vi "AlliGator Compute Pixel Phasor Array v3.vi"(6 "e^j w t_i Vector":csg[](array[numeric]), 7 "Time-Gated Reference Decay":cluster{"t Array":dbl[], "I Array":dbl[]}, 8 "Error In":errorcluster, 9 "t Array":sgl[](array[numeric]), 10 "Gate Images Stack (NxVxH)":sgl[][][](array[numeric]), 11 "Sum Image (V x H)":sgl[][](array[numeric])) -> (0 "Error Out":errorcluster, 1 "# Invalid Phasors":i32, 3 "Pixel Phasors Array (V x H)":csg[][](array[numeric]) format="%_3e", 4 "CPU (s)":dbl)   [LabVIEW 2021, in "AlliGator Phasor Plot.lvlib"]
doc: "Computes the phasor of all pixels using any user-selected decay pre-processing options."
uses:
  AlliGator Phasor Plot.lvlib
  Settings/AlliGator Settings List.ctl
  Globals, Variables, Constants/AlliGator Abort.vi
  <vilib>/Utility/error.llb/Error Cluster From Error Code.vi
  <vilib>/ErrorRing/Error Ring.xnode
  Time/Time.lvlib
  Phasor/Phasor.lvlib
  Graphs/XY Graph/XY Graph Add-Ons.lvlib
  Decay Analysis/Decay Preprocessing/AlliGator Decay Preprocessing.lvlib
  Globals, Variables, Constants/AlliGator Globals, Variables & Constants.lvlib
  Settings/AlliGator Settings.lvlib
  Error/Error.lvlib
  Utilities/Utilities.lvlib
panel:
  out "Local Error":errorcluster
  # "see the AlliGator License on the block diagram (Ctrl+E or Window:Show Block Diagram)"
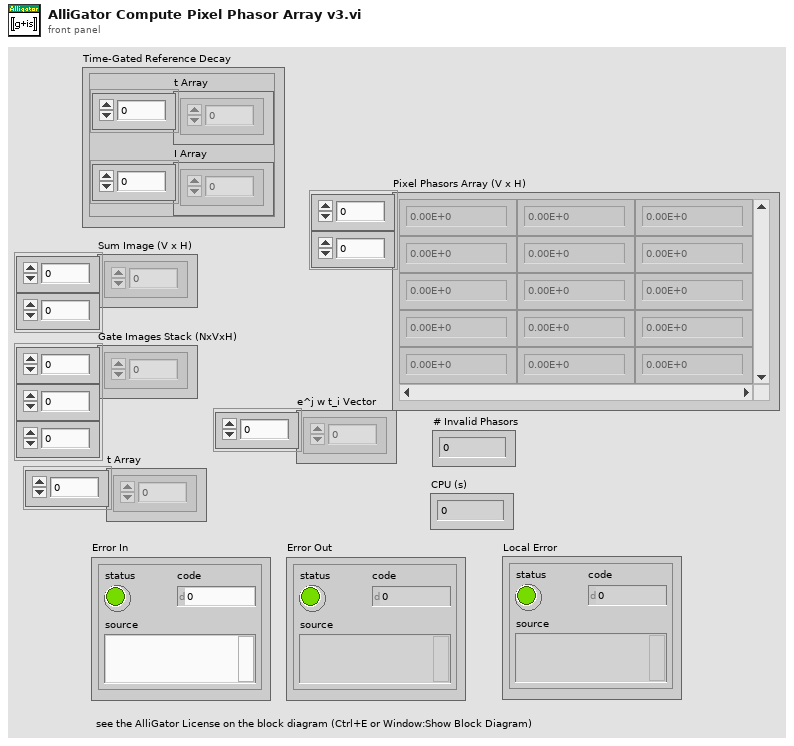
[diagram p1: front panel]
types:
  T1 = typedef "AlliGator Settings.lvlib/AlliGator Settings List.ctl" = enum16{"GUI:Visible Settings Tab", "GUI:Last Run Version", "Source Image:Use Image Histogram for Contrast", "Source Image:Low Count Pixels Rejection Options", "Source Image:High Count Pixels Rejection Options", "Source Image:Use Image Brightness", "Source Image:Blend Overlay with Image Background", "Source Image:Use Fixed ROI Diameter", "Source Image:ROI Diameter", "Source Image:ROI Center Color", "Source Image:Peak Threshold", "Source Image:Intensity Threshold", "Source Image:Image Binning Options", "Source Image:Image Smoothing Options", "Source Image:Image Histogram Active", "Source Image:Invert Binary Mask", "Source Image:Hot Pixel Removal", "Source Image:Overlay Analyzed ROI Center", "Source Image:Auto-Adjust Contrast", "Source Image:Histogram Lower Percentile", "Source Image:Histogram Upper Percentile", "Source Image:Save Source Image", "Source Image:Scale Bar Options", "Source Image:Image Resolution (Pixel Size)", "Source Image:Flatfield Correction", "Source Image:Show Dead Left Columns Correction", "Source Image:Dead Left Columns Correction", "Source Image:Image Pre-Processing Operations Order", "Source Image:Overlay ROI Median", "Source Image:Median Overlay Color", "Data Information:Gate Width", "Data Information:Nanotime Gate Separation", "Data Information:Macrotime Gate Separation", "Data Information:Gate Step", "Data Information:# Gates", "Data Information:Gate Image Exposure", "Data Information:Gate Image Integration", "Data Information:Gates to Skip", "Data Information:Gates to Keep", "Data Information:Define Gates to", "Data Information:Channel Name", "Data Information:Available Channel Names", "Data Information:Channel Arithmetic", "Data Information:Background File Subtraction", "Data Information:Background File", "Data Information:Background Scaling Factor", "Data Information:Background Pile-up Correction", "Data Information:Background Pixel Well Capacity", "Data Information:Laser Period", "Data Information:SYNC Period", "Data Information:Pile-up Correction", "Data Information:Pixel Well Capacity", "Data Information:Dataset Scaling Factor", "Fluorescence Decay_Decay Pre-Processing:Reverse Gates", "Fluorescence Decay_Decay Pre-Processing:Verbose Decay Pre-Processing", "Fluorescence Decay_Decay Pre-Processing:Use Decay Pre-Processing", "Fluorescence Decay_Decay Pre-Processing:Background Subtraction", "Fluorescence Decay_Decay Pre-Processing:Background Definition Range", "Fluorescence Decay_Decay Pre-Processing:Baseline Subtraction Method", "Fluorescence Decay_Decay Pre-Processing:Decay Pre-Processing Operations Order", "Fluorescence Decay_Decay Pre-Processing:Smoothing Parameter", "Fluorescence Decay_Decay Pre-Processing:Shift Decay", "Fluorescence Decay_Decay Pre-Processing:Decay Shift Parameters", "Fluorescence Decay_Decay Pre-Processing:Fold Decay", "Fluorescence Decay_Decay Pre-Processing:# Folds", "Fluorescence Decay_Decay Pre-Processing:1-Normalize Decay", "Fluorescence Decay_Decay Pre-Processing:[0-1]-Normalize Decay", "Fluorescence Decay_Decay Pre-Processing:Smoothen Decay", "Fluorescence Decay_Decay Pre-Processing:Extrapolate Decay", "Fluorescence Decay_Decay Pre-Processing:Use Periodicity", "Fluorescence Decay_Decay Pre-Processing:Use Cursors", "Fluorescence Decay_Decay Pre-Processing:Tail Fraction", "Fluorescence Decay_Decay Pre-Processing:Head Fraction", "Fluorescence Decay_Decay Pre-Processing:Additional Points", "Fluorescence Decay_Decay Pre-Processing:Straighten Decay", "Fluorescence Decay_Decay Pre-Processing:Constant Background", "Fluorescence Decay_Decay Pre-Processing:Pixel-Normalize Decay", "Fluorescence Decay_Advanced Analysis:Extract IRF instead of Decay", "Fluorescence Decay_Advanced Analysis:IRF Extraction Options", "Fluorescence Decay_Advanced Analysis:IRF Optimization Options", "Fluorescence Decay_Advanced Analysis:Square Pulse Options", "Fluorescence Decay_Advanced Analysis:IRF Order", "Fluorescence Decay_Advanced Analysis:IRF Time Constants", "Fluorescence Decay_Advanced Analysis:Wavelet Analysis Options", "Fluorescence Decay_Advanced Analysis:Average Lifetime Options", "Fluorescence Decay_Fit Options:Fit Options", "Fluorescence Decay_Fit Options:Use Legacy Fitting Approach", "Fluorescence Decay_Fit Options:Use Data Information Laser Period", "Fluorescence Decay_Fit Parameters:Displayed Fit Parameters", "Fluorescence Decay_Fit Parameters:Fit Parameter Constraints", "Fluorescence Decay_Fit Parameters:Export Tabulated Results", "Fluorescence Decay_Fit Parameters:MLE Baseline Offset Type", "Fluorescence Decay_Fit Parameters:MLE Baseline Offset", "Fluorescence Decay_Fit Parameters:Guess Parameter Names", "Fluorescence Decay_Fit Parameters:Guess Parameter Values", "Fluorescence Decay_Fit Parameters:Guess Parameters Options", "Fluorescence Decay_Fit Parameters:Optimal Offset Selection Criterion", "Fluorescence Decay_Styles:Show Last Decay Only", "Fluorescence Decay_Styles:Decay Graph Color Array", "Fluorescence Decay:Decay Graph Active", "Fluorescence Decay Statistics:Min Peak Value", "Fluorescence Decay Statistics:Reject Low Decay Peak Pixels", "Fluorescence Decay Statistics:Reject High Decay Peak Pixels", "Fluorescence Decay Statistics:Max Peak Value", "Time Traces:Use File Timestamp", "Time Traces:Time Step", "Time Traces:Use Intensity Correction File", "Time Traces:Intensity Correction File", "Phasor Plot:Phasor Plot Smoothing Options", "Phasor Plot:Phasor Plot Size", "Phasor Plot:Phasor Plot Graphics Options", "Phasor Plot:Cumulative Phasor Plot", "Phasor Plot:Use Phasor Brightness", "Phasor Plot:Blend Overlay with Phasor Background", "Phasor Plot:Save Phasor Plot", "Phasor Plot:Show References", "Phasor Plot:Phasor Ratio Decay Range", "Phasor Plot:Exponential Fading", "Phasor Plot:Phasor Ratio Reference Colors", "Phasor Plot:Reference Radius", "Phasor Plot:Show Color Map Vertices", "Phasor Plot:Phasor Plot Active", "Phasor Plot:Phasor Ratio Color Map Type", "Phasor Plot:Phasor Ratio Color Map", "Phasor Plot:Phasor Ratio Display Range", "Phasor Plot:Selected Image ROI(s)", "Phasor Plot:All Image ROIs", "Phasor Plot:Selected Phasor Plot ROI(s)", "Phasor Plot:All Phasor Plot ROIs", "Phasor Plot:Phasor Ratio Color-Coded Quantity", "Phasor Plot:Store Phasor Harmonics", "Phasor Plot:Draw Reference Segment", "Phasor Plot:User-Defined Quantity", "Phasor Plot:Color Scale High Color", "Phasor Plot:Color Scale Low Color", "Phasor Graph:Phasor Frequency", "Phasor Graph:Phasor Ratio Type", "Phasor Graph:Pixel-level Phasor Computation", "Phasor Graph:Save Phasor Graph", "Phasor Graph:Phasor Graph Active", "Phasor Graph:Phasor SDV Options", "Phasor Calibration:Use Backup Calibration if needed", "Phasor Graph:Define Shortest Lifetime as", "Phasor Calibration:Backup Calibration Type", "Phasor Calibration:Calibration Type", "Phasor Calibration:Calibration Lifetime", "Phasor Calibration:Calibration Map Algorithm", "Single-Exponential Phasor Locus (SEPL):Gate Parameters", "Single-Exponential Phasor Locus (SEPL):User-defined Gate", "Single-Exponential Phasor Locus (SEPL):User-defined IRF", "Single-Exponential Phasor Locus (SEPL):Phasor Parameters", "Single-Exponential Phasor Locus (SEPL):Decay & IRF Parameters", "Single-Exponential Phasor Locus (SEPL):Display Parameters", "Lifetime Analysis:Decay Analysis Parameters", "Lifetime Analysis:Lifetime Map Active", "Plugins:Python Settings", "Miscellaneous:Verbose Mode", "Miscellaneous:Beep after Script", "Miscellaneous:Saved Image File Format", "Miscellaneous:Exported Gate Image Settings", "Miscellaneous:Include Loading in Timing", "Miscellaneous:Verbose Settings Mode", "Miscellaneous:Histogram Options", "Miscellaneous:Beep on Error", "Miscellaneous:# Logical Processors Used", "Miscellaneous:ROI Description Max Characters", "Miscellaneous:Verbose Error Mode", "Miscellaneous:Transparent Mask Color"}
  T2 = typedef "AlliGator Decay Preprocessing.lvlib/AlliGator Decay Preprocessing Options.ctl" = cluster{"Background Subtraction Parameters":T3, "Decay Preprocessing Parameters":T5, "Preprocessing Steps Order":string[]}
  T3 = typedef "AlliGator Decay Preprocessing.lvlib/AlliGator Background Subtraction Parameters.ctl" = cluster{"Background Definition Range":cluster{"Min Gate":dbl[unit], "Max Gate":dbl[unit]}, "Baseline Subtraction Method":T4, "Background Subtraction?":bool, "Background File":path, "Background Constant":dbl, "Background Scaling Factor":dbl, "Background Pile-up Correction":bool, "Background Pixel Well Capacity":u32}
  T4 = typedef "AlliGator Decay Preprocessing.lvlib/AlliGator Baseline Subtraction Method.ctl" = enum16{"Mean", "Min", "Square Gated Single-Exponential", "File", "Constant"}
  T5 = typedef "AlliGator Decay Preprocessing.lvlib/AlliGator Decay Preprocessing Parameters.ctl" = cluster{"Background Subtraction":bool, "Straighten Decay":bool, "Reverse Gates":bool, "1-Normalized Decay":bool, "Smoothen Decay":bool, "Smoothing Parameter":dbl, "Shift Decay":bool, "Decay Shift Parameters":T6, "Extrapolate Decay":bool, "Additional Points":u32, "Head Fraction":dbl, "Pixel-Normalize Decay":bool, "Use Periodicity":bool, "Use Cursors":bool, "Tail Fraction":dbl, "Use Decay Pre-Processing":bool, "Fold Decay":bool, "# Folds":u32, "[0-1]-Normalized Decay":bool}
  T6 = typedef "XY Graph Add-Ons.lvlib/XY Graph Plot Shift Parameters.ctl" = cluster{"Type":T7, "Shift":dbl[unit], "Threshold":dbl, "Rotate":bool}
  T7 = typedef "XY Graph Add-Ons.lvlib/XY Graph Plot Shift Method.ctl" = enum16{"Default", "CFD", "Threshold", "Cross-Correlation"}
  T8 = cluster{"Min Gate":dbl[unit], "Max Gate":dbl[unit]}
  T9 = cluster{"t Axis":dbl[], "ROI Intensity Array in":dbl[]}
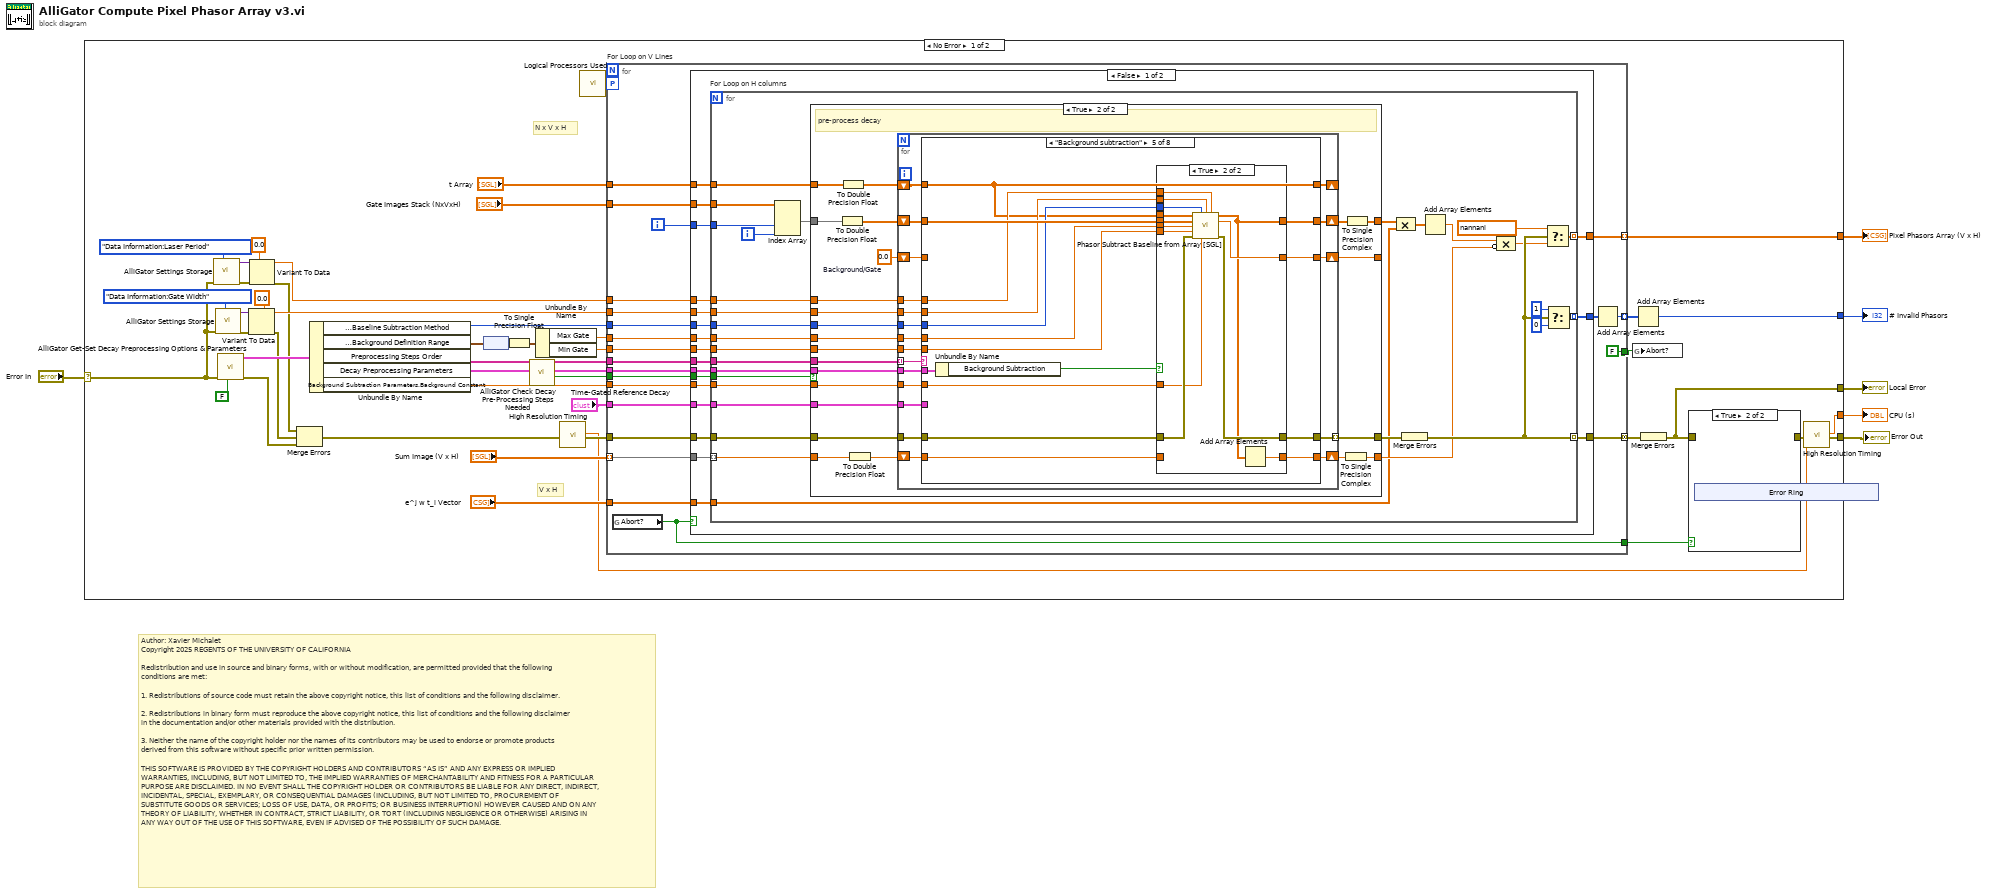
[diagram p0: block diagram]
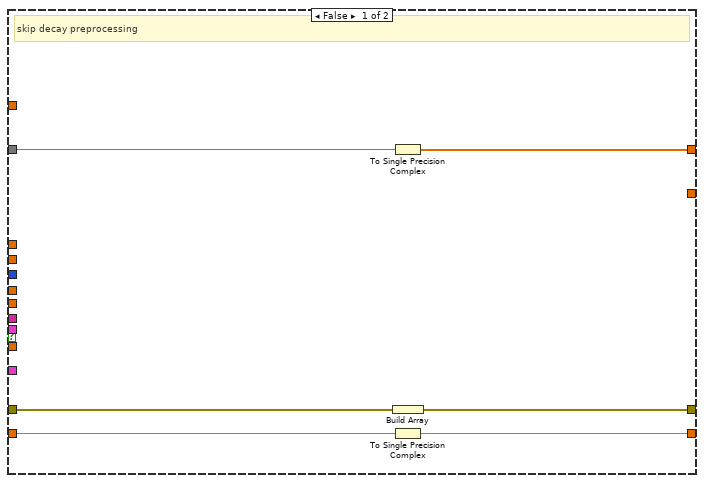
[diagram p2: hidden frame]
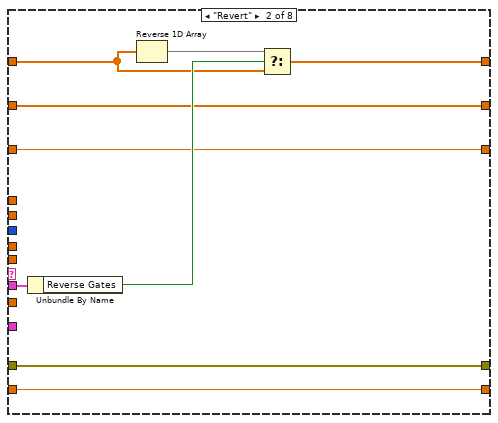
[diagram p4: hidden frame]
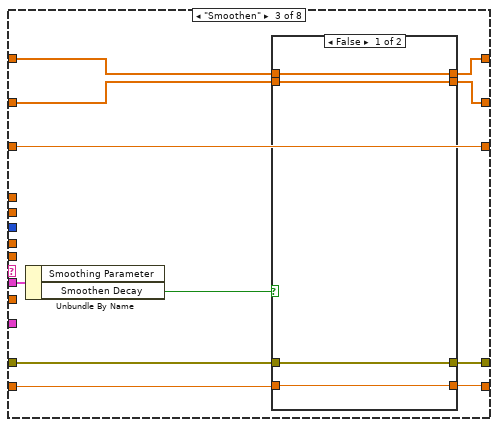
[diagram p5: hidden frame]
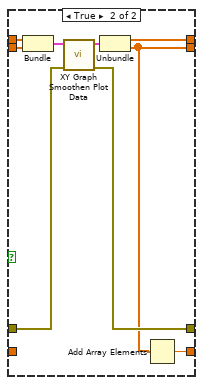
[diagram p6: hidden frame]
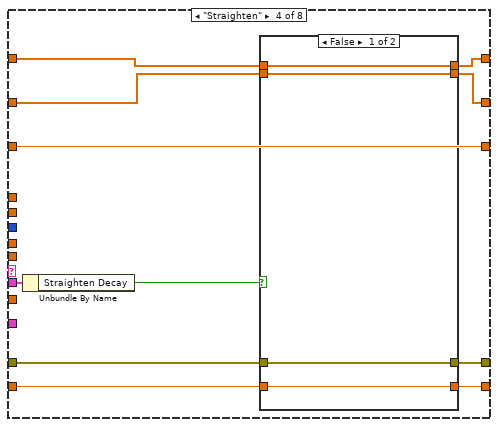
[diagram p7: hidden frame]
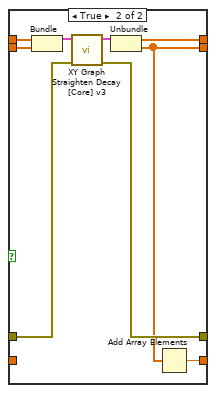
[diagram p8: hidden frame]
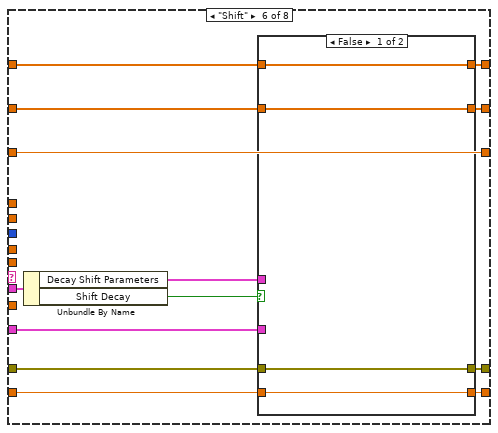
[diagram p10: hidden frame]
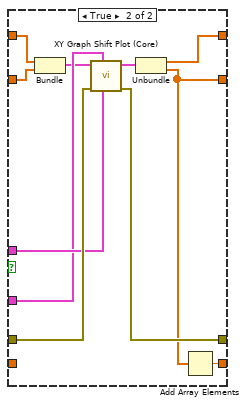
[diagram p11: hidden frame]
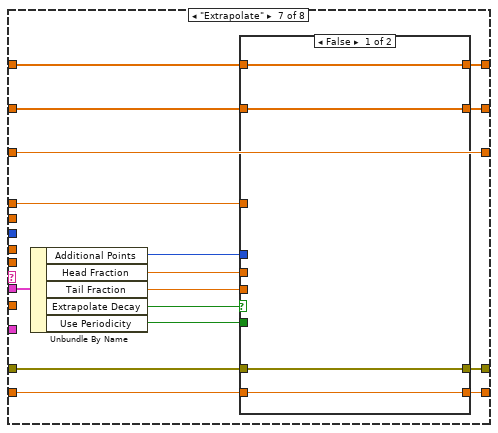
[diagram p12: hidden frame]
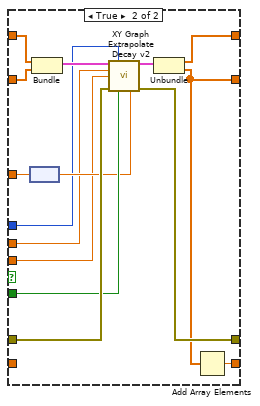
[diagram p13: hidden frame]
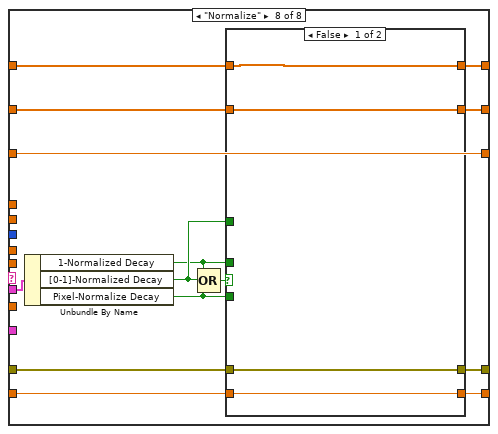
[diagram p14: hidden frame]
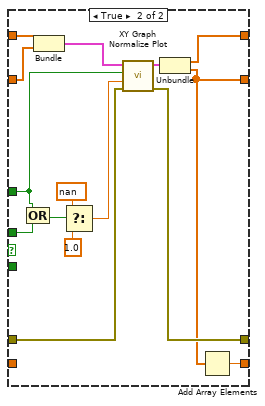
[diagram p15: hidden frame]
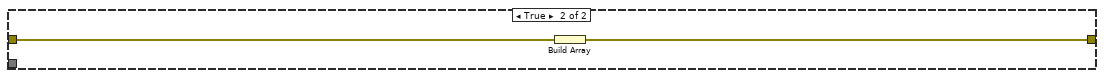
[diagram p16: hidden frame]
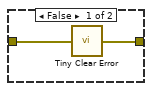
[diagram p17: hidden frame]
diagram:
  # "Author: Xavier Michalet\nCopyright 2025 REGENTS OF THE UNIVERSITY OF CALIFORNIA\n\nRedistribution and use in source and binary forms, with or without modification, are permitted provided that the following conditions are met:\n\n1. Redistributions of source code must retain the above copyright notice, this list of conditions and the following disclaimer.\n\n2. Redistributions in binary form must reproduce the above copyright notice, this list of conditions and the following disclaimer in the documentation and/or other materials provided with the distribution.\n\n3. Neither the name of the copyright holder nor the names of its contributors may be used to endorse or promote products derived from this software without specific prior written permission.\n\nTHIS SOFTWARE IS PROVIDED BY THE COPYRIGHT HOLDERS AND CONTRIBUTORS “AS IS” AND ANY EXPRESS OR IMPLIED WARRANTIES, INCLUDING, BUT NOT LIMITED TO, THE IMPLIED WARRANTIES OF MERCHANTABILITY AND FITNESS FOR A PARTICULAR PURPOSE ARE DISCLAIMED. IN NO EVENT SHALL THE COPYRIGHT HOLDER OR CONTRIBUTORS BE LIABLE FOR ANY DIRECT, INDIRECT, INCIDENTAL, SPECIAL, EXEMPLARY, OR CONSEQUENTIAL DAMAGES (INCLUDING, BUT NOT LIMITED TO, PROCUREMENT OF SUBSTITUTE GOODS OR SERVICES; LOSS OF USE, DATA, OR PROFITS; OR BUSINESS INTERRUPTION) HOWEVER CAUSED AND ON ANY THEORY OF LIABILITY, WHETHER IN CONTRACT, STRICT LIABILITY, OR TORT (INCLUDING NEGLIGENCE OR OTHERWISE) ARISING IN ANY WAY OUT OF THE USE OF THIS SOFTWARE, EVEN IF ADVISED OF THE POSSIBILITY OF SUCH DAMAGE."
  n1 = case shown="No Error" "Error In" {
    selector: "Error In" -> [w18 w371]
    tunnel: [w49 _] -> w6
    tunnel: [w48 _] -> w5
    tunnel: [w47 w371] -> w4
    tunnel: [w16 _] -> w2
    tunnel: [w15 _] -> w1
    frame No Error {
      # "V x H"
      # "N x V x H"
      n2 = call "AlliGator Settings Storage.vi"("AlliGator Settings List"=AlliGator_Settings_List."Data Information:Laser Period", "Error In"=w18) -> ("Error Out"=w30:errorcluster, "Variant Data out"=w31:variant)  [unwired: 8 in]
      n3 = call "AlliGator Settings Storage.vi"("AlliGator Settings List"=AlliGator_Settings_List."Data Information:Gate Width", "Error In"=w18) -> ("Error Out"=w20:errorcluster, "Variant Data out"=w29:variant)  [unwired: 8 in]
      n4 = call "AlliGator Get-Set Decay Preprocessing Options & Parameters.vi"("Get (F)/Set"=FALSE, "error in (no error)"=w18) -> ("error out"=w41:errorcluster, "Decay Preprocessing Options & Parameters out"=w35:T2)  [unwired: 8 in]
      n5 = Variant To Data(error in=w20, type=dbl[unit] 0.0 ("Laser Period"), Variant=w29) -> (data=w24:dbl[unit], error out=w22:errorcluster)
      n6 = Variant To Data(error in=w30, type=dbl[unit] 0.0 ("Laser Period"), Variant=w31) -> (data=w25:dbl[unit], error out=w21:errorcluster)
      n7 = Merge Errors(w21, w22, w41) -> (w23:errorcluster)
      n8 = Unbundle By Name(w35) -> ("Background Subtraction Parameters.Baseline Subtraction Method"=w34:T4, "Background Subtraction Parameters.Background Definition Range"=w33:T8, "Preprocessing Steps Order"=w13:string[], "Decay Preprocessing Parameters"=w12:T5, "Background Subtraction Parameters.Background Constant"=w14:dbl)
      n9 = node(w33) -> (w43:cluster{"Min Gate":dbl, "Max Gate":dbl})
      n10 = To Single Precision Float(number=w43) -> (single precision float=w42:cluster{"Min Gate":sgl, "Max Gate":sgl})
      n11 = call "AlliGator Check Decay Pre-Processing Steps Needed.vi"("Decay Preprocessing Parameters"=w12, "Preprocessing Steps Order in"=w13) -> ("Preprocessing needed?"=w9:bool, "Decay Preprocessing Parameters (dup)"=w10:T5, "Preprocessing Steps Order out"=w11:string[])  [unwired: 7 in]
      n12 = Unbundle By Name(w42) -> ("Max Gate"=w51:sgl, "Min Gate"=w50:sgl)
      n13 = call "High Resolution Timing.vi"("Error In"=w23) -> ("elapsed (relative) seconds"=w37:dbl, "Error Out"=w40:errorcluster)  [unwired: 16 in, 1 out]
      n14 = call "Logical Processors Used.vi"() -> ("# Logical Processor Used"=w7:i32)  [unwired: 6 in]
      n15 = for "For Loop on V Lines" {
        tunnel: "Gate Images Stack (NxVxH)" -> [w75]
        tunnel: "e^j w t_i Vector" -> [w74]
        tunnel: "Sum Image (V x H)" -> [w73] mode=indexing
        tunnel: [w71] -> w49 mode=indexing
        tunnel: "t Array" -> [w70]
        tunnel: w51 -> [w69]
        tunnel: w50 -> [w68]
        tunnel: w34 -> [w67]
        tunnel: w24 -> [w66]
        tunnel: w25 -> [w65]
        tunnel: [w56] -> w44
        tunnel: w40 -> [w64]
        tunnel: [w63] -> w39 mode=concatenating
        tunnel: "Time-Gated Reference Decay" -> [w62]
        tunnel: w11 -> [w61]
        tunnel: w10 -> [w60]
        workers-P: w7 -> [_]
        tunnel: [FALSE ("Abort?")] -> w19
        tunnel: [w57] -> w17 mode=indexing
        tunnel: w14 -> [w55]
        tunnel: w9 -> [w54]
        i -> [w72]
        n16 = global read "AlliGator Abort.vi" "Abort?"() -> (w56:bool)
        n17 = case shown="False" w56 {
          tunnel: w75 -> [w94 _]
          tunnel: w74 -> [w93 _]
          tunnel: w73 -> [w92 _]
          tunnel: w72 -> [w91 _]
          tunnel: [w90 _] -> w71
          tunnel: w70 -> [w89 _]
          tunnel: w69 -> [w88 _]
          tunnel: w68 -> [w87 _]
          tunnel: w67 -> [w86 _]
          tunnel: w66 -> [w85 _]
          tunnel: w65 -> [w84 _]
          tunnel: w64 -> [w83 w363]
          tunnel: [w82 w362] -> w63
          tunnel: w62 -> [w81 _]
          tunnel: w61 -> [w80 _]
          tunnel: w60 -> [w79 _]
          tunnel: [w78 _] -> w58
          tunnel: w55 -> [w77 _]
          tunnel: w54 -> [w76 _]
          frame False {
            n18 = for "For Loop on H columns" {
              tunnel: w94 -> [w124]
              tunnel: w93 -> [w96]
              tunnel: w91 -> [w119]
              tunnel: w92 -> [w98] mode=indexing
              tunnel: [w106] -> w90 mode=indexing
              tunnel: w89 -> [w112]
              tunnel: w88 -> [w117]
              tunnel: w87 -> [w116]
              tunnel: w86 -> [w118]
              tunnel: w85 -> [w115]
              tunnel: w84 -> [w114]
              tunnel: w83 -> [w111]
              tunnel: [w104] -> w82 mode=indexing
              tunnel: w81 -> [w109]
              tunnel: w80 -> [w108]
              tunnel: w79 -> [w107]
              tunnel: [w101] -> w78 mode=indexing
              tunnel: w77 -> [w100]
              tunnel: w76 -> [w99]
              i -> [w120]
              n19 = Index Array(array=w124, index (dim 1)=w119, index (dim 2)=w120) -> (element=w121:sgl[])  [unwired: 1 in]
              n20 = case shown="True" w99 {
                tunnel: w121 -> [w130 w153]
                tunnel: w118 -> [_ w152]
                tunnel: w117 -> [_ w151]
                tunnel: w116 -> [_ w150]
                tunnel: [_ w149] -> _
                tunnel: w115 -> [_ w148]
                tunnel: w114 -> [_ w147]
                tunnel: [w126 w132] -> w113
                tunnel: w112 -> [_ w144]
                tunnel: w111 -> [w129 w143]
                tunnel: [w128 w142] -> w110
                tunnel: w109 -> [_ w141]
                tunnel: w108 -> [_ w140]
                tunnel: w107 -> [_ w139]
                tunnel: w100 -> [_ w138]
                tunnel: w98 -> [w127 w137]
                tunnel: [w125 w131] -> w97
                frame False {
                  # "skip decay preprocessing"
                  n21 = To Single Precision Complex(1:w130) -> (0:w126:csg[])
                  n22 = Build Array(w129) -> (w128:errorcluster[])
                  n23 = To Single Precision Complex(1:w127) -> (0:w125:csg)
                }
                frame True {
                  w146 = 0.0  # Background/Gate
                  # "pre-process decay"
                  n24 = To Double Precision Float(number=w153) -> (double precision float=w134:dbl[])
                  n25 = To Double Precision Float(number=w144) -> (double precision float=w135:dbl[])
                  n26 = To Double Precision Float(number=w137) -> (double precision float=w133:dbl)
                  n27 = for {
                    tunnel: w152 -> [w171]
                    tunnel: w151 -> [w170]
                    tunnel: w150 -> [w169]
                    tunnel: w148 -> [w167]
                    tunnel: w147 -> [w166]
                    shift-right: [w168] -> w149
                    shift-left: w146 -> [w165]
                    shift-right: [w164] -> w145
                    shift-left: w134 -> [w172]
                    shift-right: [w162] -> _
                    shift-left: w135 -> [w163]
                    tunnel: w143 -> [w161]
                    tunnel: [w160] -> w142 mode=indexing
                    tunnel: w141 -> [w159]
                    tunnel: w140 -> [w158] mode=indexing
                    tunnel: w139 -> [w157]
                    tunnel: w138 -> [w156]
                    shift-right: [w154] -> w136
                    shift-left: w133 -> [w155]
                    n28 = case shown="\"Background subtraction\"" w158 {
                      tunnel: w163 -> [w176 w185 w194 w219 w241 w273 w305 w339]
                      tunnel: w172 -> [w175 w181 w195 w218 w250 w271 w303 w337]
                      tunnel: [w175 w181 w192 w216 w249 w270 w302 w336] -> w164
                      tunnel: w171 -> [_ _ _ _ w248 _ _ _]
                      tunnel: w170 -> [_ _ _ _ w247 _ _ _]
                      tunnel: w169 -> [_ _ _ _ w246 _ _ _]
                      tunnel: [w177 w183 w197 w221 w245 w279 w309 w342] -> w168
                      tunnel: w167 -> [_ _ _ _ w244 _ _ _]
                      tunnel: w166 -> [_ _ _ _ w243 _ w297 _]
                      tunnel: w165 -> [w177 w183 w197 w221 _ w279 w309 w342]
                      tunnel: [w176 w182 w193 w217 w241 w272 w304 w338] -> w162
                      tunnel: w161 -> [w174 w180 w191 w215 w240 w275 w307 w341]
                      tunnel: [w174 w180 w190 w214 w239 w274 w306 w340] -> w160
                      tunnel: w159 -> [_ _ _ _ _ w276 _ _]
                      tunnel: w157 -> [_ w179 w189 w213 w238 w269 w300 w335]
                      tunnel: w156 -> [_ _ _ _ w237 _ _ _]
                      tunnel: w155 -> [w173 w178 w188 w212 w236 w267 w295 w333]
                      tunnel: [w173 w178 w187 w211 w235 w268 w296 w332] -> w154
                      frame Default {
                      }
                      frame "Revert" {
                        n29 = Unbundle By Name(w179) -> ("Reverse Gates"=w186:bool)
                        n30 = Reverse 1D Array(array=w185) -> (reversed array=w184:dbl[])
                        n31 = Select(t=w184, s=w186, f=w185) -> (s? t:f=w182:dbl[])
                      }
                      frame "Smoothen" {
                        n32 = Unbundle By Name(w189) -> ("Smoothen Decay"=w196:bool)  [unwired: 1 out]
                        n33 = case shown="False" w196 {
                          tunnel: w194 -> [w201 w210]
                          tunnel: w195 -> [w200 w209]
                          tunnel: [w201 w206] -> w193
                          tunnel: [w200 w203] -> w192
                          tunnel: w191 -> [w199 w205]
                          tunnel: [w199 w204] -> w190
                          tunnel: w188 -> [w198 _]
                          tunnel: [w198 w202] -> w187
                          frame False {
                          }
                          frame True {
                            n34 = Bundle(w210, w209) -> (w208:cluster{dbl[], dbl[]})  [unwired: 1 in]
                            n35 = call "XY Graph Smoothen Plot Data.vi"("Error In"=w205, "Plot"=w208) -> ("error out"=w204:errorcluster, "Cubic Splined Plot"=w207:cluster{"X Array":dbl[], "Y Array":dbl[]})  [unwired: 8 in]
                            n36 = Unbundle(w207) -> ("X Array"=w206:dbl[], "Y Array"=w203:dbl[])
                            n37 = Add Array Elements(numeric array=w203) -> (sum=w202:dbl)
                          }
                        }
                      }
                      frame "Straighten" {
                        n38 = Unbundle By Name(w213) -> ("Straighten Decay"=w220:bool)
                        n39 = case shown="False" w220 {
                          tunnel: w219 -> [w225 w234]
                          tunnel: w218 -> [w224 w233]
                          tunnel: [w225 w230] -> w217
                          tunnel: [w224 w227] -> w216
                          tunnel: w215 -> [w223 w229]
                          tunnel: [w223 w228] -> w214
                          tunnel: w212 -> [w222 _]
                          tunnel: [w222 w226] -> w211
                          frame False {
                          }
                          frame True {
                            n40 = Bundle(w234, w233) -> (w232:cluster{dbl[], dbl[]})  [unwired: 1 in]
                            n41 = call "XY Graph Straighten Decay [Core] v3.vi"("Error In"=w229, "Plot in"=w232) -> ("error out"=w228:errorcluster, "Plot out"=w231:cluster{"X Array":dbl[], "Y Array":dbl[]})  [unwired: 7 in, 1 out]
                            n42 = Unbundle(w231) -> ("X Array"=w230:dbl[], "Y Array"=w227:dbl[])
                            n43 = Add Array Elements(numeric array=w227) -> (sum=w226:dbl)
                          }
                        }
                      }
                      frame "Background subtraction" {
                        n44 = Unbundle By Name(w238) -> ("Background Subtraction"=w242:bool)
                        n45 = case shown="True" w242 {
                          tunnel: w241 -> [_ w266]
                          tunnel: w250 -> [w253 w265]
                          tunnel: [w253 w255] -> w249
                          tunnel: w248 -> [_ w264]
                          tunnel: w247 -> [_ w263]
                          tunnel: w246 -> [_ w262]
                          tunnel: [_ w261] -> w245
                          tunnel: w244 -> [_ w260]
                          tunnel: w243 -> [_ w259]
                          tunnel: w240 -> [w252 w258]
                          tunnel: [w252 w257] -> w239
                          tunnel: w237 -> [_ w256]
                          tunnel: w236 -> [w251 _]
                          tunnel: [w251 w254] -> w235
                          frame False {
                          }
                          frame True {
                            n46 = call "Phasor Subtract Baseline from Array [SGL].vi"("X Array"=w266, "Method (Min)"=w264, "Gate Duration"=w260, "Laser Period"=w259, "Y Array"=w265, "Max X"=w263, "Min X"=w262, "Error In"=w258, "Background Constant"=w256) -> ("Bkgd-subtracted Y Array"=w255:sgl[], "Background/Gate"=w261:sgl, "Error Out"=w257:errorcluster)  [unwired: 1 in, 3 out]
                            n47 = Add Array Elements(numeric array=w255) -> (sum=w254:sgl)
                          }
                        }
                      }
                      frame "Shift" {
                        n48 = Unbundle By Name(w269) -> ("Decay Shift Parameters"=w277:T6, "Shift Decay"=w278:bool)
                        n49 = case shown="False" w278 {
                          tunnel: w277 -> [_ w292]
                          tunnel: w276 -> [_ w291]
                          tunnel: w275 -> [w283 w294]
                          tunnel: [w283 w293] -> w274
                          tunnel: w273 -> [w282 w290]
                          tunnel: [w282 w286] -> w272
                          tunnel: w271 -> [w281 w289]
                          tunnel: [w281 w285] -> w270
                          tunnel: [w280 w284] -> w268
                          tunnel: w267 -> [w280 _]
                          frame False {
                          }
                          frame True {
                            n50 = Bundle(w290, w289) -> (w288:cluster{dbl[], dbl[]})  [unwired: 1 in]
                            n51 = call "XY Graph Shift Plot (Core).vi"("Plot Shift Parameters"=w292, "Time-Gated Reference Decay"=w291, "error in (no error)"=w294, "Decay in"=w288) -> ("error out"=w293:errorcluster, "Decay out"=w287:T9)  [unwired: 5 in, 1 out]
                            n52 = Unbundle(w287) -> ("t Axis"=w286:dbl[], "ROI Intensity Array in"=w285:dbl[])
                            n53 = Add Array Elements(numeric array=w285) -> (sum=w284:dbl)
                          }
                        }
                      }
                      frame "Extrapolate" {
                        n54 = Unbundle By Name(w300) -> ("Additional Points"=w301:u32, "Head Fraction"=w298:dbl, "Extrapolate Decay"=w308:bool, "Use Periodicity"=w299:bool)  [unwired: 1 out]
                        n55 = case shown="False" w308 {
                          tunnel: w307 -> [w313 w328]
                          tunnel: [w313 w327] -> w306
                          tunnel: w305 -> [w312 w326]
                          tunnel: [w312 w322] -> w304
                          tunnel: w303 -> [w311 w325]
                          tunnel: [w311 w315] -> w302
                          tunnel: w298 -> [_ w317]
                          tunnel: w301 -> [_ w318]
                          tunnel: w299 -> [_ w321]
                          tunnel: w297 -> [_ w320]
                          tunnel: w298 -> [_ w316]
                          tunnel: [w310 w314] -> w296
                          tunnel: w295 -> [w310 _]
                          frame False {
                          }
                          frame True {
                            n56 = node(w320) -> (w319:dbl)
                            n57 = Bundle(w326, w325) -> (w324:cluster{dbl[], dbl[]})  [unwired: 1 in]
                            n58 = call "XY Graph Extrapolate Decay v2.vi"("Plot in"=w324, "# Additional Points (-1: to Period)"=w318, "Head Fraction"=w316, "Tail Fraction"=w317, "Error In"=w328, "Periodic Decay"=w321, "Period"=w319) -> ("Plot out"=w323:cluster{"X Array":dbl[], "Y Array":dbl[]}, "error out"=w327:errorcluster)  [unwired: 3 in, 4 out]
                            n59 = Unbundle(w323) -> ("X Array"=w322:dbl[], "Y Array"=w315:dbl[])
                            n60 = Add Array Elements(numeric array=w315) -> (sum=w314:dbl)
                          }
                        }
                      }
                      frame "Normalize" {
                        n61 = Unbundle By Name(w335) -> ("1-Normalized Decay"=w329:bool, "[0-1]-Normalized Decay"=w331:bool, "Pixel-Normalize Decay"=w330:bool)
                        n62 = Compound Arithmetic op=OR(w329, w331, w330) -> (w334:bool)
                        n63 = case shown="False" w334 {
                          tunnel: w341 -> [w346 w361]
                          tunnel: [w346 w360] -> w340
                          tunnel: w339 -> [w344 w359]
                          tunnel: [w344 w355] -> w338
                          tunnel: w337 -> [w345 w358]
                          tunnel: [w345 w351] -> w336
                          tunnel: w333 -> [w343 _]
                          tunnel: [w343 w350] -> w332
                          tunnel: w331 -> [_ w349]
                          tunnel: w330 -> [_ _]
                          tunnel: w329 -> [_ w348]
                          frame False {
                          }
                          frame True {
                            n64 = Compound Arithmetic op=OR(w349, w348) -> (w347:bool)
                            n65 = Bundle(w359, w358) -> (w357:cluster{dbl[], dbl[]})  [unwired: 1 in]
                            n66 = Select(t=nan ("Normalization Factor"), s=w347, f=1.0) -> (s? t:f=w352:dbl)
                            n67 = call "XY Graph Normalize Plot.vi"("Error In"=w361, "Normalization Factor (Max *)"=w352, "Subtract Baseline? (No)"=w349, "Plot in"=w357) -> ("Error Out"=w360:errorcluster, "Plot out"=w356:cluster{"X Array":dbl[], "Y Array":dbl[]})  [unwired: 6 in]
                            n68 = Unbundle(w356) -> ("X Array"=w355:dbl[], "Y Array"=w351:dbl[])
                            n69 = Add Array Elements(numeric array=w351) -> (sum=w350:dbl)
                          }
                        }
                      }
                    }
                  }
                  n70 = To Single Precision Complex(1:w136) -> (0:w131:csg)
                  n71 = To Single Precision Complex(1:w145) -> (0:w132:csg[])
                }
              }
              n72 = Compound Arithmetic op=MULTIPLY(w113, w96) -> (w123:csg[])
              n73 = Merge Errors(w110) -> (w104:errorcluster)
              n74 = Add Array Elements(numeric array=w123) -> (sum=w122:csg)
              n75 = Compound Arithmetic op=MULTIPLY(w122, invert w97) -> (w95:csg)
              n76 = Select(t=csg nan+nani, s=w104, f=w95) -> (s? t:f=w106:csg)
              n77 = Select(t=1, s=w104, f=0) -> (s? t:f=w101:i32)
            }
          }
          frame True {
            n78 = Build Array(w363) -> (w362:errorcluster[])
          }
        }
        n79 = Add Array Elements(numeric array=w58) -> (sum=w57:i32)
      }
      n80 = global write "AlliGator Abort.vi" "Abort?"(w19) -> ()
      n81 = Add Array Elements(numeric array=w17) -> (sum=w16:i32)
      n82 = Merge Errors(w39) -> (w15:errorcluster)
      n83 = case shown="True" w44 {
        tunnel: [w364 w366] -> w38
        tunnel: w15 -> [w365 _]
        frame False {
          n84 = call "Tiny Clear Error.vi"("Error In"=w365) -> ("no Error Out"=w364:errorcluster)  [unwired: 8 in]
        }
        frame True {
          n85 = xnode "Error Ring"() -> ("error out"=w366:errorcluster)
        }
      }
      n86 = call "High Resolution Timing.vi"("relative seconds (NaN)"=w37, "Error In"=w38) -> ("elapsed (relative) seconds"=w48:dbl, "Error Out"=w47:errorcluster)  [unwired: 15 in, 1 out]
    }
    frame Error {
    }
  }
  "Pixel Phasors Array (V x H)" <- w6
  "Error Out" <- w4
  "CPU (s)" <- w5
  "# Invalid Phasors" <- w2
  "Local Error" <- w1
